vi "ParseBS.vi"(11 "BS String":string) -> (1 "Y Pos":dbl, 2 "X Pos":dbl, 3 "Target Locations":dbl[][](array[numeric]))   [LabVIEW 2012]
panel:
  out "String":string
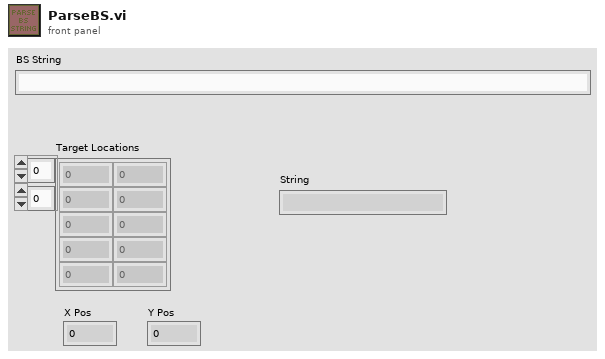
[diagram p1: front panel]
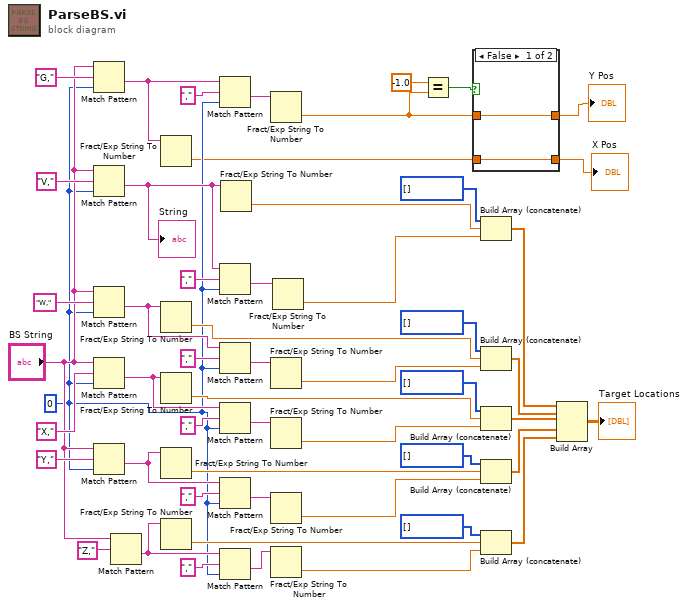
[diagram p0: block diagram]
diagram:
  w7 = 0 ("offset (0)")
  n1 = Match Pattern(string="BS String", regular expression="G,", offset (0)=w7) -> (after substring=w17:string)  [unwired: 3 out]
  n2 = Match Pattern(string="BS String", regular expression="V,", offset (0)=w7) -> (after substring=w43:string)  [unwired: 3 out]
  "String" <- w43
  n3 = Match Pattern(string="BS String", regular expression="W,", offset (0)=w7) -> (after substring=w42:string)  [unwired: 3 out]
  n4 = Match Pattern(string="BS String", regular expression="X,", offset (0)=w7) -> (after substring=w32:string)  [unwired: 3 out]
  n5 = Match Pattern(string="BS String", regular expression="Y,", offset (0)=w7) -> (after substring=w29:string)  [unwired: 3 out]
  n6 = Match Pattern(string="BS String", regular expression="Z,") -> (after substring=w13:string)  [unwired: 1 in, 3 out]
  n7 = Fract/Exp String To Number(string=w17) -> (number=w2:dbl)  [unwired: 3 in, 1 out]
  n8 = Fract/Exp String To Number(string=w42) -> (number=w35:dbl)  [unwired: 3 in, 1 out]
  n9 = Fract/Exp String To Number(string=w32) -> (number=w26:dbl)  [unwired: 3 in, 1 out]
  n10 = Fract/Exp String To Number(string=w29) -> (number=w24:dbl)  [unwired: 3 in, 1 out]
  n11 = Fract/Exp String To Number(string=w13) -> (number=w12:dbl)  [unwired: 3 in, 1 out]
  n12 = Match Pattern(string=w17, regular expression=",", offset (0)=w7) -> (after substring=w18:string)  [unwired: 3 out]
  n13 = Match Pattern(string=w43, regular expression=",", offset (0)=w7) -> (after substring=w44:string)  [unwired: 3 out]
  n14 = Match Pattern(string=w42, regular expression=",", offset (0)=w7) -> (after substring=w47:string)  [unwired: 3 out]
  n15 = Match Pattern(string=w32, regular expression=",", offset (0)=w7) -> (after substring=w48:string)  [unwired: 3 out]
  n16 = Match Pattern(string=w29, regular expression=",", offset (0)=w7) -> (after substring=w30:string)  [unwired: 3 out]
  n17 = Match Pattern(string=w13, regular expression=",", offset (0)=w7) -> (after substring=w14:string)  [unwired: 3 out]
  n18 = Fract/Exp String To Number(string=w43) -> (number=w40:dbl)  [unwired: 3 in, 1 out]
  n19 = Fract/Exp String To Number(string=w18) -> (number=w6:dbl)  [unwired: 3 in, 1 out]
  n20 = Fract/Exp String To Number(string=w47) -> (number=w34:dbl)  [unwired: 3 in, 1 out]
  n21 = Fract/Exp String To Number(string=w48) -> (number=w25:dbl)  [unwired: 3 in, 1 out]
  n22 = Fract/Exp String To Number(string=w30) -> (number=w23:dbl)  [unwired: 3 in, 1 out]
  n23 = Fract/Exp String To Number(string=w14) -> (number=w11:dbl)  [unwired: 3 in, 1 out]
  n24 = Fract/Exp String To Number(string=w44) -> (number=w39:dbl)  [unwired: 3 in, 1 out]
  n25 = Equal?(x=-1.0, y=w6) -> (x = y?=w4:bool)
  n26 = case shown="False" w4 {
    tunnel: w6 -> [w55 _]
    tunnel: [w55 _] -> w3
    tunnel: w2 -> [w54 _]
    tunnel: [w54 _] -> w1
    frame False {
    }
    frame True {
    }
  }
  "X Pos" <- w1
  "Y Pos" <- w3
  n27 = Build Array (concatenate)(i32[] [], w40, w39) -> (w38:dbl[])
  n28 = Build Array (concatenate)(i32[] [], w35, w34) -> (w33:dbl[])
  n29 = Build Array (concatenate)(i32[] [], w26, w25) -> (w22:dbl[])
  n30 = Build Array (concatenate)(i32[] [], w24, w23) -> (w21:dbl[])
  n31 = Build Array (concatenate)(i32[] [], w12, w11) -> (w9:dbl[])
  n32 = Build Array(w38, w33, w22, w21, w9) -> (→"Target Locations":dbl[][])
